vi "shgnoref.vi"() -> ()   [LabVIEW 2020]
uses:
  <vilib>/DAQmx/read.llb/DAQmx Read (Counter 1D U32 1Chan NSamp).vi
  <vilib>/DAQmx/create/channels.llb/DAQmx Create Channel (CI-Period).vi
  <vilib>/DAQmx/configure/timing.llb/DAQmx Timing (Implicit).vi
  <vilib>/DAQmx/create/channels.llb/DAQmx Create Channel (CO-Pulse Generation-Frequency).vi
  <vilib>/DAQmx/miscellaneous.llb/DAQmx Fill In Error Info.vi
  <resource>/objmgr/daqmx.rc
  <vilib>/Analysis/NI_AALBase.lvlib
panel:
  out "mean":dbl(graph)
  out "Numeric Indicator":dbl
  in  "samples per loop ref":i32=1
  out "Ref. Channel":dbl(graph)
  out "Waveform Chart 2":dynamicdata(graph)
  out "Waveform Chart":u32[](graph)
  in  "stop":bool
  out "count":u32[](array[numeric])
  in  "samples per loop":i32=1
  in  "dwell time (ms)":dbl=1.0 format="%.6f"
  in  "Photon Input (PFI)":tag="/Dev1/PFI0"
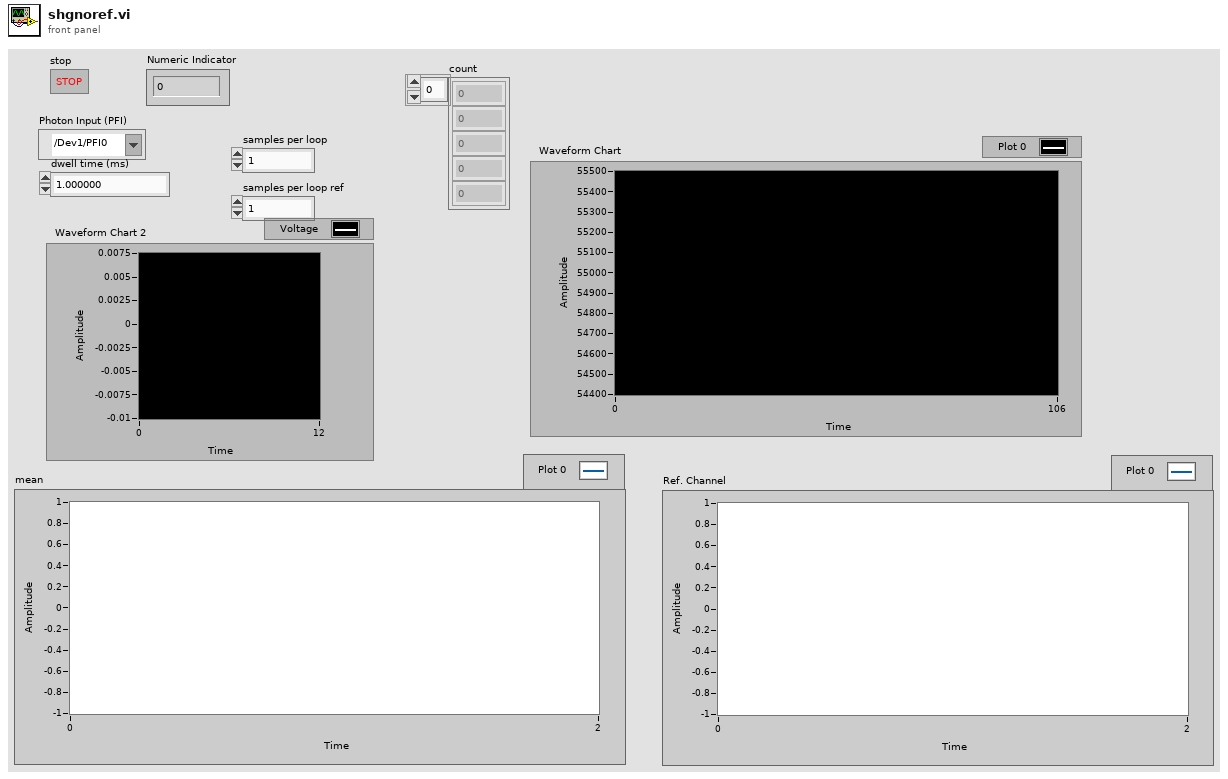
[diagram p1: front panel]
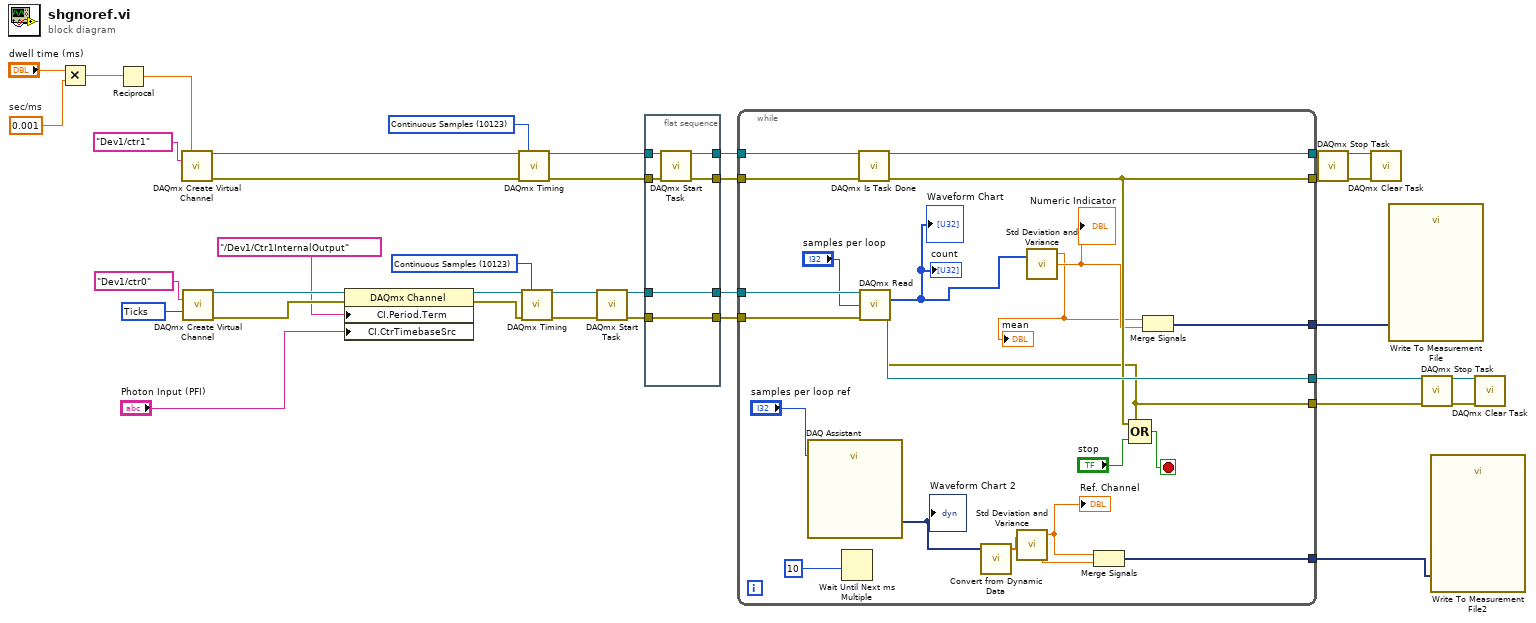
[diagram p0: block diagram]
diagram:
  w9 = 0.001  # sec/ms
  w19 = 10304 items=["Seconds"=10364, "Ticks"=10304, "From Custom Scale"=10065] ("units")
  w20 = 10123 items=["Finite Samples"=10178, "Continuous Samples"=10123, "Hardware Timed Single Point"=12522] ("sample mode")
  w21 = 10123 items=["Finite Samples"=10178, "Continuous Samples"=10123, "Hardware Timed Single Point"=12522] ("sample mode")
  n1 = Multiply(x="dwell time (ms)", y=w9) -> (x*y=w8:dbl)
  n2 = Reciprocal(x=w8) -> (1/x=w7:dbl)
  n3 = call-poly <vilib>:"DAQmx Create Virtual Channel.vi"("frequency"=w7, "counter"=tag "Dev1/ctr1") -> ("task out"=w36:refnum<k21>, "error out"=w37:errorcluster)  [unwired: 12 in]
  n4 = call-poly <vilib>:"DAQmx Create Virtual Channel.vi"("counter"=tag "Dev1/ctr0", "units"=w19) -> ("task out"=w16:refnum<k21>, "error out"=w15:errorcluster)  [unwired: 12 in]
  n5 = property class="DAQmx Channel"(reference=w16, error in=w15, "CI.Period.Term"=tag "/Dev1/Ctr1InternalOutput", "CI.CtrTimebaseSrc"="Photon Input (PFI)") -> (reference out=w14:refnum<k21>, error out=w13:errorcluster)
  n6 = call-poly <vilib>:"DAQmx Timing.vi"("task/channels in"=w36, "sample mode"=w21, "error in"=w37) -> ("task out"=w35:refnum<k21>, "error out"=w34:errorcluster)  [unwired: 11 in]
  n7 = call-poly <vilib>:"DAQmx Timing.vi"("task/channels in"=w14, "sample mode"=w20, "error in"=w13) -> ("task out"=w27:refnum<k21>, "error out"=w26:errorcluster)  [unwired: 11 in]
  n8 = call <vilib>:"DAQmx Start Task.vi"("task/channels in"=w27, "error in"=w26) -> ("task out"=w5:refnum<k21>, "error out"=w3:errorcluster)  [unwired: 12 in]
  n9 = flat-sequence {
    tunnel: w35 -> [w43]
    tunnel: w34 -> [w42]
    tunnel: [w41] -> w33
    tunnel: [w40] -> w32
    tunnel: [w39] -> w6
    tunnel: w5 -> [w39]
    tunnel: [w38] -> w4
    tunnel: w3 -> [w38]
    frame #0 {
      n10 = call <vilib>:"DAQmx Start Task.vi"("task/channels in"=w43, "error in"=w42) -> ("task out"=w40:refnum<k21>, "error out"=w41:errorcluster)  [unwired: 12 in]
    }
  }
  n11 = while {
    tunnel: w33 -> [w65]
    tunnel: w32 -> [w64]
    tunnel: [w57] -> w31
    tunnel: [w63] -> w30
    tunnel: [w62] -> w25
    tunnel: [w56] -> w24
    tunnel: w6 -> [w61]
    tunnel: w4 -> [w60]
    tunnel: [w45] -> w2
    tunnel: [w44] -> w1
    stop <- w55 stop-if-true
    n12 = call "DAQ Assistant"("number of samples"="samples per loop ref") -> ("data"=w54:dynamicdata)  [unwired: 16 in, 2 out]
    "Waveform Chart 2" <- w54
    n13 = Wait Until Next ms Multiple(millisecond multiple=10) -> ()  [unwired: 1 out]
    n14 = call <vilib>:"DAQmx Is Task Done.vi"("task/channels in"=w64, "error in"=w65) -> ("task out"=w63:refnum<k21>, "error out"=w57:errorcluster)  [unwired: 11 in, 1 out]
    n15 = call-poly <vilib>:"DAQmx Read.vi"("task/channels in"=w61, "number of samples per channel"="samples per loop", "error in"=w60) -> ("task out"=w62:refnum<k21>, "data"=w49:u32[], "error out"=w56:errorcluster)  [unwired: 10 in]
    "count" <- w49
    "Waveform Chart" <- w49
    n16 = call "Convert from Dynamic Data"("Dynamic Data Type"=w54) -> ("Array"=w53:dbl[])  [unwired: 3 in]
    n17 = call <vilib>:"Std Deviation and Variance.vi"("X"=w53) -> ("mean"=w52:dbl, "standard deviation"=w51:dbl)  [unwired: 1 in, 1 out]
    "Ref. Channel" <- w52
    n18 = call <vilib>:"Std Deviation and Variance.vi"("X"=w49) -> ("mean"=w46:dbl, "standard deviation"=w47:dbl)  [unwired: 1 in, 1 out]
    "Numeric Indicator" <- w47
    "mean" <- w46
    n19 = Merge Signals(w52, w51) -> (w44:dynamicdata)
    n20 = Compound Arithmetic op=OR(w57, w56, "stop") -> (w55:bool)
    n21 = Merge Signals(w46, w47) -> (w45:dynamicdata)
  }
  n22 = call <vilib>:"DAQmx Stop Task.vi"("task/channels in"=w30, "error in"=w31) -> ("task out"=w29:refnum<k21>, "error out"=w28:errorcluster)  [unwired: 12 in]
  n23 = call <vilib>:"DAQmx Clear Task.vi"("task in"=w29, "error in"=w28) -> ()  [unwired: 13 in, 1 out]
  n24 = call "Write To Measurement File"("Signals"=w2) -> ()  [unwired: 16 in, 3 out]
  n25 = call <vilib>:"DAQmx Stop Task.vi"("task/channels in"=w25, "error in"=w24) -> ("task out"=w22:refnum<k21>, "error out"=w23:errorcluster)  [unwired: 12 in]
  n26 = call "Write To Measurement File2"("Signals"=w1) -> ()  [unwired: 16 in, 3 out]
  n27 = call <vilib>:"DAQmx Clear Task.vi"("task in"=w22, "error in"=w23) -> ()  [unwired: 13 in, 1 out]
